vi "fgv_UI-dev-operator.vi"(7 "cmd":T1, 8 "error in (no error)":errorcluster) -> (0 "error out":errorcluster)   [LabVIEW 2019]
uses:
  UI dev-operator.ctl
  _ctrl/rw.ctl
  SubVIs/common/Glob_Ref.vi
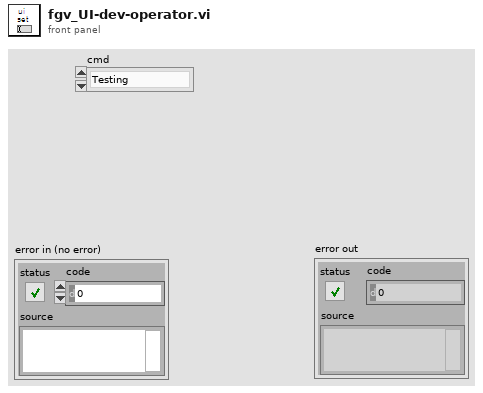
[diagram p1: front panel]
types:
  T1 = typedef "UI dev-operator.ctl" = enum16{"Testing", "Admin", "Operator", "Finish", "Ready"}
  T2 = typedef "rw.ctl" = enum16{"read", "write"}
  T3 = typedef "ui_dev-operator.ctl" = cluster{"Operation stutus":refnum<vi>, "Test Status":refnum<vi>, "Setting":refnum<vi>, "Manual":refnum<vi>, "Main":refnum<vi>, "RCstart":refnum<vi>, "채널선택":refnum<vi>, "시험명":refnum<vi>, "Tab Control_manual":refnum<vi>, "시험 모드":refnum<vi>, "HW check":refnum<vi>, "login":refnum<vi>, "logout":refnum<vi>}
  T4 = typedef "ref_all.ctl" = cluster{"BP4610 Config":refnum<vi>, "DSP1950 Config":refnum<vi>, "2470-config":refnum<vi>, "cDAQ 9269 AO config":refnum<vi>, "cDAQ 9221 Config":refnum<vi>, "cDAQ-9467 Config":refnum<vi>, "Waveform":refnum<vi>, "DL950 wfm":refnum<vi>, "AI Graph":refnum<vi>, "AO_Wave-config":refnum<vi>, "DL950 items":refnum<vi>, "Volt":refnum<vi>, "Current":refnum<vi>, "AO_Level":refnum<vi>, "RC-Test Judgement ":refnum<vi>, "Log path":refnum<vi>, "시험명":refnum<vi>, "file renew[Hr]":refnum<vi>, "Breakdown-Spec":refnum<vi>, "paste":refnum<vi>, "copy":refnum<vi>, "DL950_config":refnum<vi>, "종료시간":refnum<vi>, "경과시간":refnum<vi>, "Apply":refnum<vi>, "DSP Config LV ":refnum<vi>, "Testconfig":refnum<vi>}
  T5 = enum8{"Enabled", "Disabled", "Disabled and Grayed Out"}
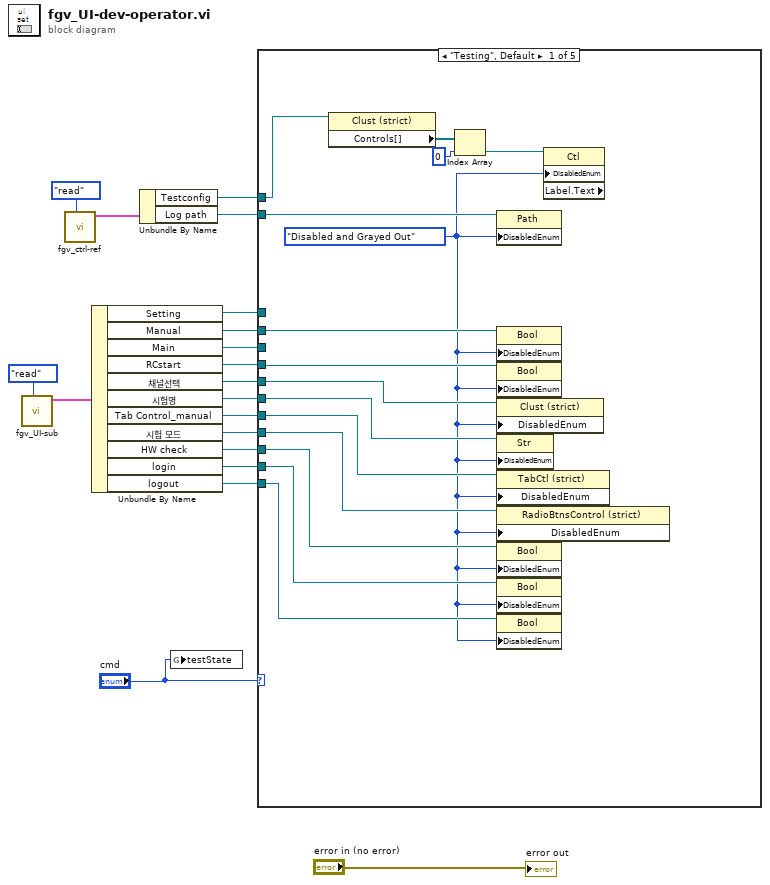
[diagram p0: block diagram]
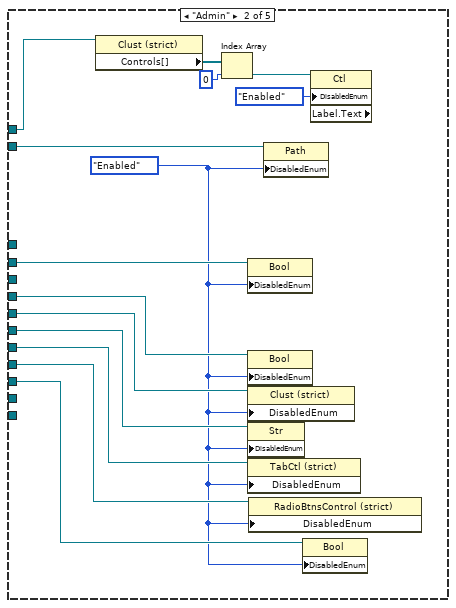
[diagram p2: hidden frame]
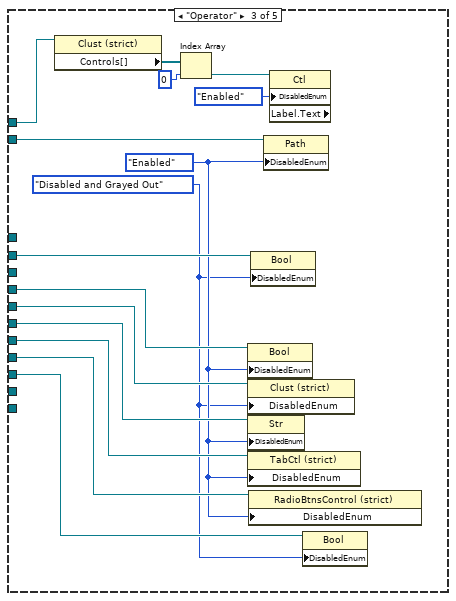
[diagram p3: hidden frame]
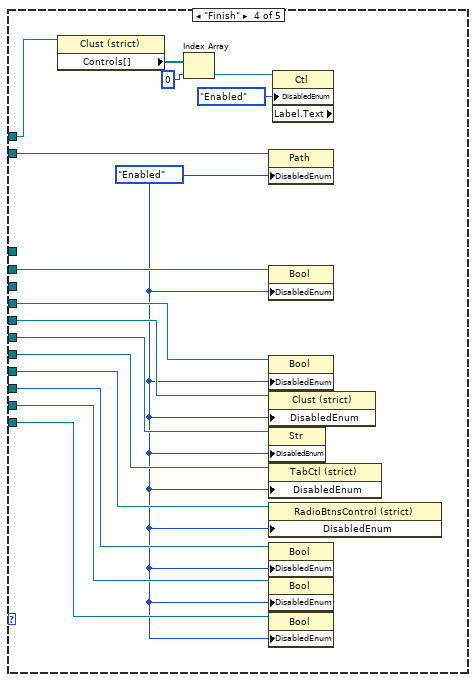
[diagram p4: hidden frame]
diagram:
  n1 = call "fgv_UI-sub.vi"("cmd"=rw."read") -> ("output cluster 2"=w18:T3)  [unwired: 9 in, 1 out]
  n2 = call "fgv_ctrl-ref.vi"("cmd"=rw."read") -> ("output cluster 2"=w8:T4)  [unwired: 9 in, 1 out]
  n3 = Unbundle By Name(w18) -> ("Setting"=w17:refnum<vi>, "Manual"=w16:refnum<vi>, "Main"=w15:refnum<vi>, "RCstart"=w14:refnum<vi>, "채널선택"=w13:refnum<vi>, "시험명"=w12:refnum<vi>, "Tab Control_manual"=w11:refnum<vi>, "시험 모드"=w10:refnum<vi>, "HW check"=w4:refnum<vi>, "login"=w3:refnum<vi>, "logout"=w2:refnum<vi>)
  n4 = Unbundle By Name(w8) -> ("Testconfig"=w1:refnum<vi>, "Log path"=w7:refnum<vi>)
  n5 = global write "Glob_Ref.vi" "testState"("cmd") -> ()
  n6 = case shown="\"Testing\", Default" "cmd" {
    tunnel: w17 -> [_ _ _ _ _]
    tunnel: w16 -> [w34 w48 w63 w79 _]
    tunnel: w15 -> [_ _ _ _ _]
    tunnel: w14 -> [w33 w47 w62 w78 _]
    tunnel: w13 -> [w32 w46 w61 w77 _]
    tunnel: w12 -> [w31 w45 w60 w76 _]
    tunnel: w11 -> [w30 w44 w59 w75 _]
    tunnel: w10 -> [w29 w43 w58 w74 _]
    tunnel: w7 -> [w28 w42 w57 w73 _]
    tunnel: w4 -> [w27 w41 w56 w72 _]
    tunnel: w3 -> [w26 _ _ w71 _]
    tunnel: w2 -> [w25 _ _ w70 _]
    tunnel: w1 -> [w21 w35 w49 w64 _]
    frame "Testing", Default {
      w20 = T5."Disabled and Grayed Out" ("Disabled")
      n7 = property class="Clust (strict)"(reference=w21) -> ("Controls[]"=w23:refnum<vi>[])  [unwired: 1 in, 2 out]
      n8 = Index Array(array=w23, index=0) -> (element=w24:refnum<vi>)
      n9 = property class="Path"(reference=w28, "DisabledEnum"=w20) -> ()  [unwired: 1 in, 2 out]
      n10 = property class="Bool"(reference=w34, "DisabledEnum"=w20) -> ()  [unwired: 1 in, 2 out]
      n11 = property class="Bool"(reference=w33, "DisabledEnum"=w20) -> ()  [unwired: 1 in, 2 out]
      n12 = property class="Clust (strict)"(reference=w32, "DisabledEnum"=w20) -> ()  [unwired: 1 in, 2 out]
      n13 = property class="Str"(reference=w31, "DisabledEnum"=w20) -> ()  [unwired: 1 in, 2 out]
      n14 = property class="TabCtl (strict)"(reference=w30, "DisabledEnum"=w20) -> ()  [unwired: 1 in, 2 out]
      n15 = property class="RadioBtnsControl (strict)"(reference=w29, "DisabledEnum"=w20) -> ()  [unwired: 1 in, 2 out]
      n16 = property class="Bool"(reference=w27, "DisabledEnum"=w20) -> ()  [unwired: 1 in, 2 out]
      n17 = property class="Bool"(reference=w26, "DisabledEnum"=w20) -> ()  [unwired: 1 in, 2 out]
      n18 = property class="Bool"(reference=w25, "DisabledEnum"=w20) -> ()  [unwired: 1 in, 2 out]
      n19 = property class="Ctl" props=["DisabledEnum", "Label", "Text"](reference=w24, "DisabledEnum"=w20) -> ()  [unwired: 1 in, 3 out]
    }
    frame "Admin" {
      w40 = T5."Enabled" ("Disabled")
      n20 = property class="Clust (strict)"(reference=w35) -> ("Controls[]"=w38:refnum<vi>[])  [unwired: 1 in, 2 out]
      n21 = Index Array(array=w38, index=0) -> (element=w39:refnum<vi>)
      n22 = property class="Bool"(reference=w48, "DisabledEnum"=w40) -> ()  [unwired: 1 in, 2 out]
      n23 = property class="Bool"(reference=w47, "DisabledEnum"=w40) -> ()  [unwired: 1 in, 2 out]
      n24 = property class="Clust (strict)"(reference=w46, "DisabledEnum"=w40) -> ()  [unwired: 1 in, 2 out]
      n25 = property class="Str"(reference=w45, "DisabledEnum"=w40) -> ()  [unwired: 1 in, 2 out]
      n26 = property class="TabCtl (strict)"(reference=w44, "DisabledEnum"=w40) -> ()  [unwired: 1 in, 2 out]
      n27 = property class="RadioBtnsControl (strict)"(reference=w43, "DisabledEnum"=w40) -> ()  [unwired: 1 in, 2 out]
      n28 = property class="Path"(reference=w42, "DisabledEnum"=w40) -> ()  [unwired: 1 in, 2 out]
      n29 = property class="Bool"(reference=w41, "DisabledEnum"=w40) -> ()  [unwired: 1 in, 2 out]
      n30 = property class="Ctl" props=["DisabledEnum", "Label", "Text"](reference=w39, "DisabledEnum"=T5."Enabled" ("Disabled")) -> ()  [unwired: 1 in, 3 out]
    }
    frame "Operator" {
      w54 = T5."Disabled and Grayed Out" ("Disabled")
      w55 = T5."Enabled" ("Disabled")
      n31 = property class="Clust (strict)"(reference=w49) -> ("Controls[]"=w52:refnum<vi>[])  [unwired: 1 in, 2 out]
      n32 = Index Array(array=w52, index=0) -> (element=w53:refnum<vi>)
      n33 = property class="Bool"(reference=w62, "DisabledEnum"=w55) -> ()  [unwired: 1 in, 2 out]
      n34 = property class="Clust (strict)"(reference=w61, "DisabledEnum"=w54) -> ()  [unwired: 1 in, 2 out]
      n35 = property class="Str"(reference=w60, "DisabledEnum"=w55) -> ()  [unwired: 1 in, 2 out]
      n36 = property class="TabCtl (strict)"(reference=w59, "DisabledEnum"=w55) -> ()  [unwired: 1 in, 2 out]
      n37 = property class="RadioBtnsControl (strict)"(reference=w58, "DisabledEnum"=w55) -> ()  [unwired: 1 in, 2 out]
      n38 = property class="Bool"(reference=w63, "DisabledEnum"=w54) -> ()  [unwired: 1 in, 2 out]
      n39 = property class="Path"(reference=w57, "DisabledEnum"=w55) -> ()  [unwired: 1 in, 2 out]
      n40 = property class="Ctl" props=["DisabledEnum", "Label", "Text"](reference=w53, "DisabledEnum"=T5."Enabled" ("Disabled")) -> ()  [unwired: 1 in, 3 out]
      n41 = property class="Bool"(reference=w56, "DisabledEnum"=w54) -> ()  [unwired: 1 in, 2 out]
    }
    frame "Finish" {
      w69 = T5."Enabled" ("Disabled")
      n42 = property class="Clust (strict)"(reference=w64) -> ("Controls[]"=w67:refnum<vi>[])  [unwired: 1 in, 2 out]
      n43 = Index Array(array=w67, index=0) -> (element=w68:refnum<vi>)
      n44 = property class="Path"(reference=w73, "DisabledEnum"=w69) -> ()  [unwired: 1 in, 2 out]
      n45 = property class="Bool"(reference=w79, "DisabledEnum"=w69) -> ()  [unwired: 1 in, 2 out]
      n46 = property class="Bool"(reference=w78, "DisabledEnum"=w69) -> ()  [unwired: 1 in, 2 out]
      n47 = property class="Clust (strict)"(reference=w77, "DisabledEnum"=w69) -> ()  [unwired: 1 in, 2 out]
      n48 = property class="Str"(reference=w76, "DisabledEnum"=w69) -> ()  [unwired: 1 in, 2 out]
      n49 = property class="TabCtl (strict)"(reference=w75, "DisabledEnum"=w69) -> ()  [unwired: 1 in, 2 out]
      n50 = property class="RadioBtnsControl (strict)"(reference=w74, "DisabledEnum"=w69) -> ()  [unwired: 1 in, 2 out]
      n51 = property class="Bool"(reference=w72, "DisabledEnum"=w69) -> ()  [unwired: 1 in, 2 out]
      n52 = property class="Bool"(reference=w71, "DisabledEnum"=w69) -> ()  [unwired: 1 in, 2 out]
      n53 = property class="Bool"(reference=w70, "DisabledEnum"=w69) -> ()  [unwired: 1 in, 2 out]
      n54 = property class="Ctl" props=["DisabledEnum", "Label", "Text"](reference=w68, "DisabledEnum"=T5."Enabled" ("Disabled")) -> ()  [unwired: 1 in, 3 out]
    }
    frame "Ready" {
    }
  }
  "error out" <- "error in (no error)"
